vi "GetType.vi"(8 "error in (no error)":errorcluster, 11 "WernerReadback Msg":refnum<class "Update_Readback Msg.lvclass">) -> (0 "error out":errorcluster, 2 "Data Sample":variant, 3 "WernerReadback Msg":refnum<class "Update_Readback Msg.lvclass">)   [LabVIEW 2015, in "CS++IEFWerner.lvlib" / "Update_Readback Msg.lvclass"]
uses:
  Update_Readback Msg.lvclass
  Update_Readback Msg.lvclass/Update_Readback Msg.ctl
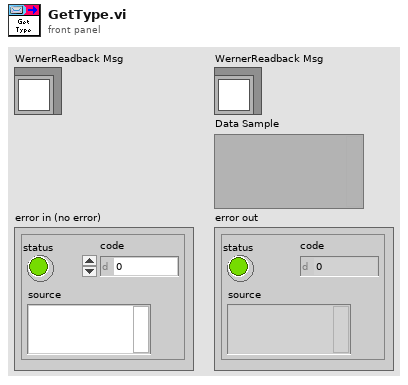
[diagram p1: front panel]
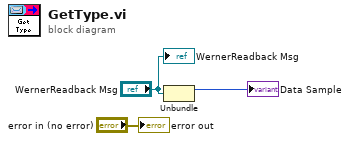
[diagram p0: block diagram]
diagram:
  n1 = Unbundle("WernerReadback Msg") -> (→"Data Sample":u32)  [unwired: 1 out]
  "error out" <- "error in (no error)"
  "WernerReadback Msg" <- "WernerReadback Msg"
